vi "Converter_calc_app-spec.vi"(0 "Data from unit number":u16, 1 "Formulas definitions":string[][](table)=[["CO ppm", "3*x"], ["O2 %", "-20*x"]], 2 "format string (app-spec file)(%f)":string="%f", 3 "enable baseline":bool, 5 "Application-specific conversion settings":T1 {"Fxn array names 2" items=[".", "O2 %", "CO ppm"]}, 7 "Legend from volts file (sensor type)":string, 9 "Value from volts file":string, 11 "error in (no error)":errorcluster, 12 "Unit's baselines for all AIs (zeros)":dbl[](array[numeric]) format="%#_13g", 13 "format string (volts file)(%f)":string="%f") -> (4 "Ledend suffix to add":string, 6 "Converted number":string, 15 "error out":errorcluster)   [LabVIEW 2013]
uses:
  Converter_app_spec_set.ctl
  <vilib>/gmath/NI_Gmath.lvlib
panel:
  out "y value":dbl format="%.2f"
  out "eq filled in x and b":string
  out "equation used":string
  # "Comma separated unit selection (-1 keyword for others)"
  # "A1.0"
  # "A1.1"
  # "A1.2"
  # "A1.3"
  # "A2.0"
  # "A2.1"
  # "A2.2"
  # "A2.3"
  # "A3.0"
  # "A3.1"
  # "A3.2"
  # "A3.3"
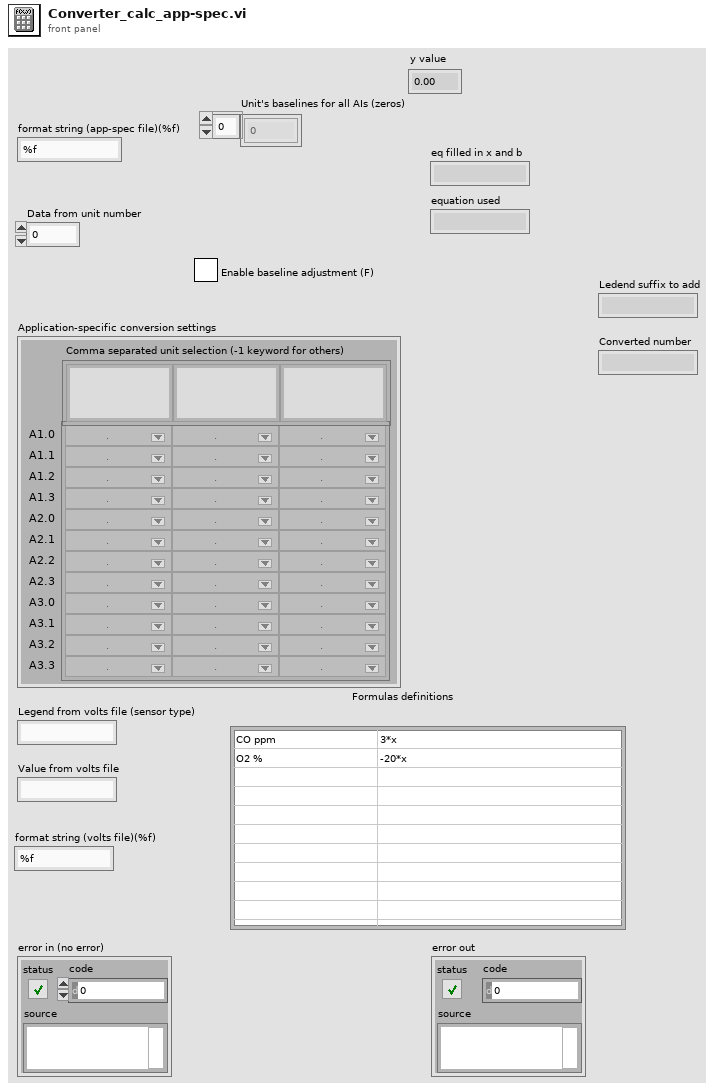
[diagram p1: front panel]
types:
  T1 = typedef "Converter_app_spec_set.ctl" = cluster{"Fxn array names 2":u16[][], "Unit conf cat. 2":string[]}
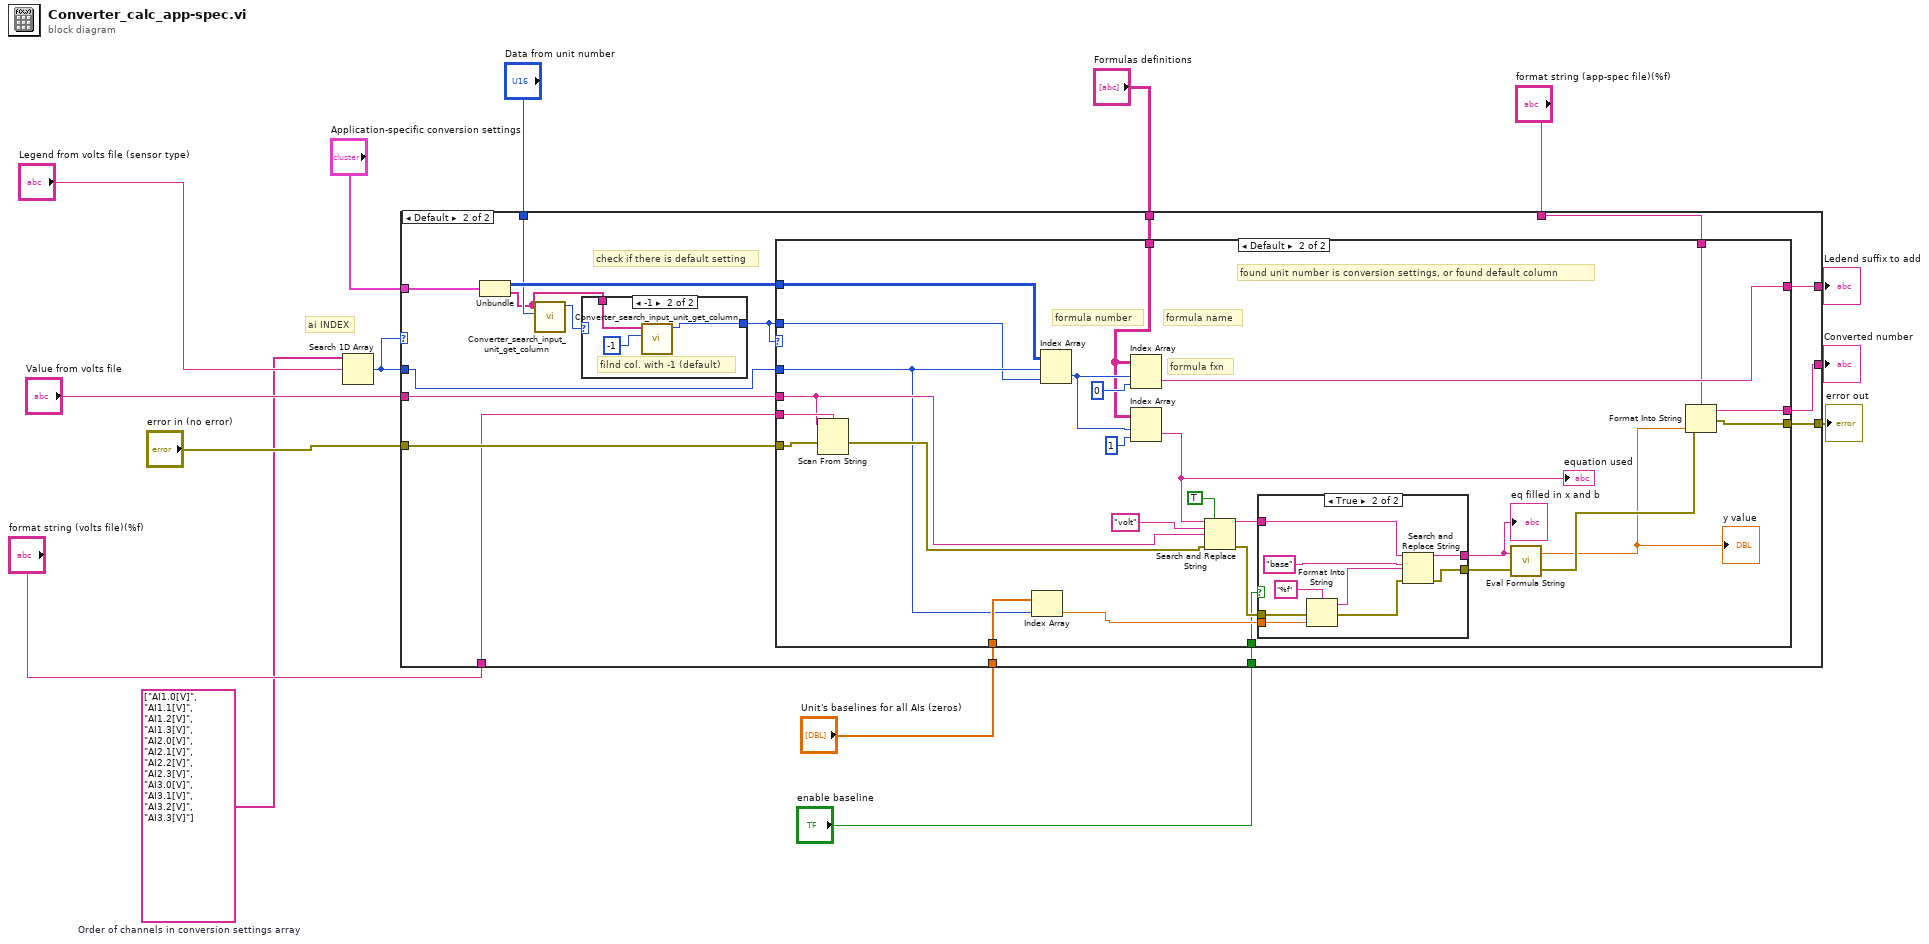
[diagram p0: block diagram]
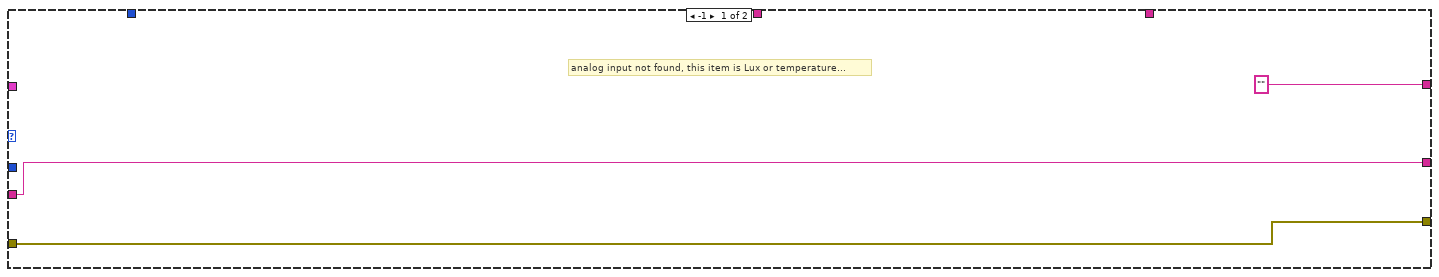
[diagram p2: hidden frame]
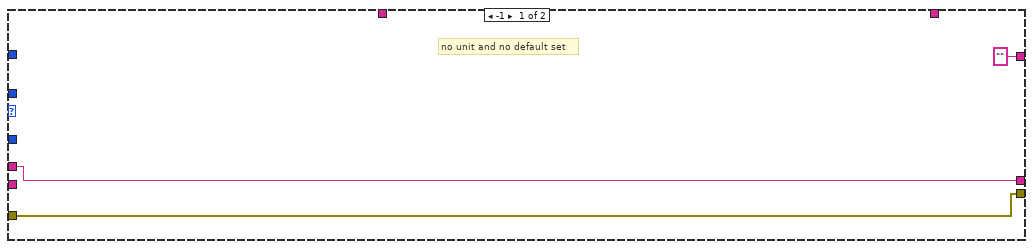
[diagram p3: hidden frame]
diagram:
  w5 = string[] ["AI1.0[V]", "AI1.1[V]", "AI1.2[V]", "AI1.3[V]", "AI2.0[V]", "AI2.1[V]", "AI2.2[V]", "AI2.3[V]", "AI3.0[V]", "AI3.1[V]", "AI3.2[V]", "AI3.3[V]"]  # Order of channels in conversion settings array
  # "ai INDEX"
  n1 = Search 1D Array(1D array=w5, element="Legend from volts file (sensor type)") -> (index of element=w3:i32)  [unwired: 1 in]
  n2 = case shown="Default" w3 {
    tunnel: "format string (volts file)(%f)" -> [_ w26]
    tunnel: "Application-specific conversion settings" -> [_ w34]
    tunnel: ["" w33] -> w13
    tunnel: w3 -> [_ w23]
    tunnel: "Data from unit number" -> [_ w32]
    tunnel: "error in (no error)" -> [w17 w31]
    tunnel: "Value from volts file" -> [w18 w25]
    tunnel: [w17 w30] -> w8
    tunnel: "format string (app-spec file)(%f)" -> [_ w29]
    tunnel: [w18 w28] -> w6
    tunnel: "Formulas definitions" -> [_ w27]
    tunnel: "Unit's baselines for all AIs (zeros)" -> [_ w24]
    tunnel: "enable baseline" -> [_ w19]
    frame -1 {
      # "analog input not found, this item is Lux or temperature..."
    }
    frame Default {
      # "check if there is default setting"
      n3 = Unbundle(w34) -> ("Fxn array names 2"=w35:u16[][], "Unit conf cat. 2"=w21:string[])
      n4 = call "Converter_search_input_unit_get_column.vi"("unit to search for"=w32, "Unit conf cat. in"=w21) -> ("found in column number"=w22:i32)  [unwired: 9 in]
      n5 = case shown="-1" w22 {
        selector: w22 -> [w77 _]
        tunnel: [w77 w78] -> w20
        tunnel: w21 -> [_ w80]
        frame 0, Default {
          # "found"
        }
        frame -1 {
          # "filnd col. with -1 (default)"
          n6 = call "Converter_search_input_unit_get_column.vi"("unit to search for"=-1, "Unit conf cat. in"=w80) -> ("found in column number"=w78:i32)  [unwired: 9 in]
        }
      }
      n7 = case shown="Default" w20 {
        tunnel: w35 -> [_ w65]
        tunnel: ["" w64] -> w33
        tunnel: w31 -> [w37 w60]
        tunnel: [w37 w59] -> w30
        tunnel: w29 -> [_ w58]
        tunnel: [w38 w57] -> w28
        tunnel: w27 -> [_ w56]
        tunnel: w26 -> [_ w53]
        tunnel: w25 -> [w38 w51]
        tunnel: w24 -> [_ w44]
        tunnel: w23 -> [_ w43]
        tunnel: w20 -> [_ w41]
        tunnel: w19 -> [_ w40]
        frame -1 {
          # "no unit and no default set"
        }
        frame Default {
          # "found unit number is conversion settings, or found default column"
          # "formula fxn"
          # "formula name"
          # "formula number"
          n8 = Scan From String(format string=w53, input string=w51, error in=w60) -> (error out=w52:errorcluster)  [unwired: 3 in, 2 out]
          n9 = Index Array(array=w44, index=w43) -> (element=w42:dbl)
          n10 = Index Array(array=w65, index (row)=w43, index (col)=w41) -> (element=w63:u16)
          n11 = Index Array(array=w56, index (row)=w63, index (col)=0 ("disabled index (col)")) -> (element=w64:string)
          n12 = Index Array(array=w56, index (row)=w63, index (col)=1 ("disabled index (col)")) -> (element=w55:string)
          "equation used" <- w55
          n13 = Search and Replace String(replace all?=TRUE ("replace all? (F)"), input string=w55, search string="volt", replace string=w51, error in=w52) -> (result string=w48:string, error out=w47:errorcluster)  [unwired: 3 in, 2 out]
          n14 = case shown="True" w40 {
            tunnel: w48 -> [w67 w76]
            tunnel: w47 -> [w66 w72]
            tunnel: [w66 w70] -> w46
            tunnel: [w67 w69] -> w45
            tunnel: w42 -> [_ w68]
            frame False {
            }
            frame True {
              n15 = Format Into String(format string="%f", error in=w72, w68) -> (resulting string=w73:string, error out=w71:errorcluster)  [unwired: 1 in]
              n16 = Search and Replace String(input string=w76, search string="base", replace string=w73, error in=w71) -> (result string=w69:string, error out=w70:errorcluster)  [unwired: 4 in, 2 out]
            }
          }
          "eq filled in x and b" <- w45
          n17 = call <vilib>:"Eval Formula String.vi"("error in (no error)"=w46, "formula"=w45) -> ("error out"=w50:errorcluster, "y value"=w49:dbl)
          "y value" <- w49
          n18 = Format Into String(format string=w58, error in=w50, w49) -> (resulting string=w57:string, error out=w59:errorcluster)  [unwired: 1 in]
        }
      }
    }
  }
  "Ledend suffix to add" <- w13
  "error out" <- w8
  "Converted number" <- w6
